vi "Correct Taus.vi"(4 "#_shots":i32=5, 6 "Filter?":bool, 8 "error in":errorcluster, 9 "filter changed?":bool, 11 "CRDS Cell in":refnum<class "CRDS Cell.lvclass">) -> (0 "error out":errorcluster, 3 "CRDS Cell out":refnum<class "CRDS Cell.lvclass">)   [LabVIEW 2014, in "CRDS Lib.lvlib" / "CRDS Cell.lvclass"]
doc: "Correct tau values for Rayleigh scattering. \n\nIf on filter:\n* The tau and tau0 values will be the uncorrected values in seconds.\n* tau0corr will be in the Rayleigh scattering corrected value in us.\n* ext, extcorr and taucorr will be set to NaN.\n\nIf on sample:\n* Tau is the raw tau value in us.\n* taucorr will be the Rayleigh scattering corrected value in us\n* ext and extCorr will be the same value."
uses:
  CRDS Cell.lvclass
  CRDS Cell.lvclass/CRDS Cell.ctl
  Data/Cell/CRDS Cell Data.lvclass/CRDS Cell Data.ctl
  Data/Cell/Read extParam.vi
  General/Atmospheric/Atmospheric Constants.vi
  Data/Cell/Read hkParam.vi
  General/Atmospheric/Atmospheric Library.lvlib
  Data/Cell/CRDS Cell Data.lvclass
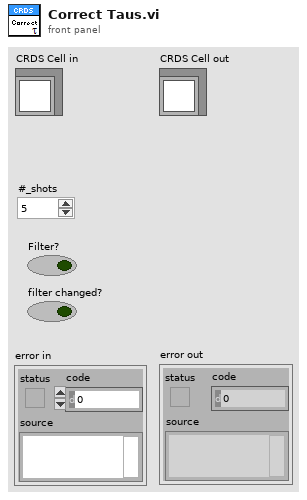
[diagram p1: front panel]
types:
  T1 = typedef "Base CRDS Lib.lvlib/calData.ctl" = cluster{"rhDilFac":sgl, "Q":sgl, "Tmean":sgl, "extDilFac":sgl, "rhCell":sgl, "P":sgl, "T":sgl}
  T2 = typedef "extparam.ctl" = cluster{"Tau":sgl, "Tau0cor":sgl, "ext":sgl, "extCorr":sgl, "stdevTau":sgl, "eTau":sgl, "taucorr":sgl, "Tau0":sgl, "max":sgl}
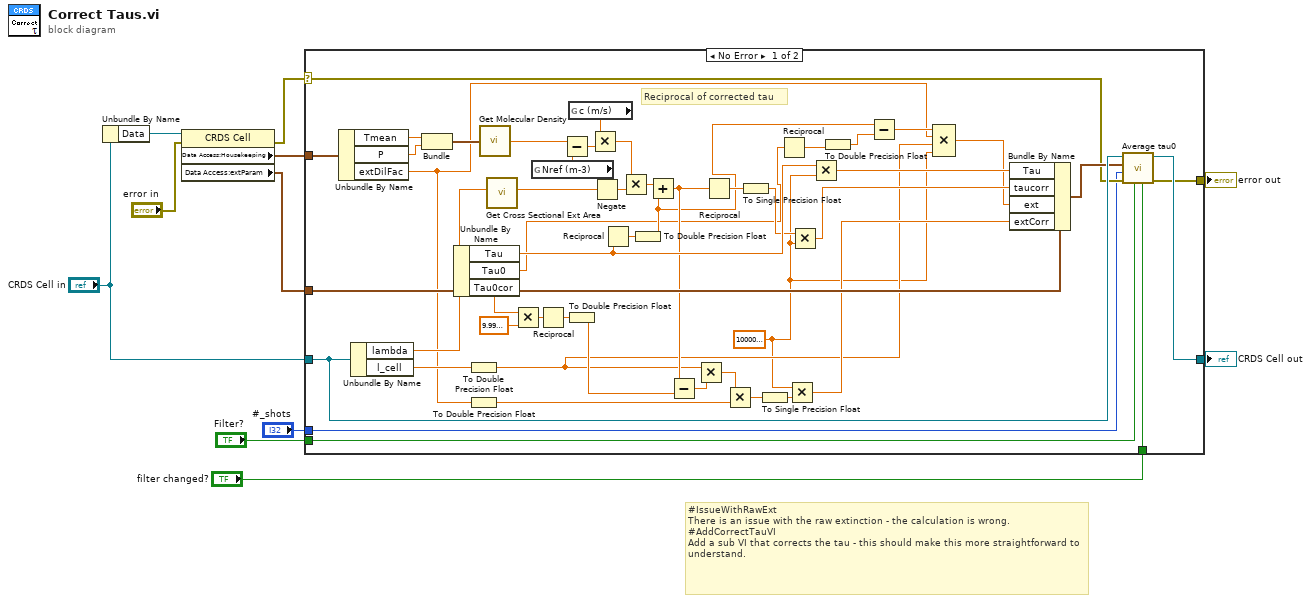
[diagram p0: block diagram]
diagram:
  # "#IssueWithRawExt\nThere is an issue with the raw extinction - the calculation is wrong.\n#AddCorrectTauVI\nAdd a sub VI that corrects the tau - this should make this more straightforward to understand."
  n1 = Unbundle By Name("CRDS Cell in") -> ("Data"=w4:refnum<class "CRDS Cell Data.lvclass">)
  n2 = property class="CRDS Cell"(reference=w4, error in="error in") -> (error out=w6:errorcluster, "Data Access:Housekeeping"=w9:T1, "Data Access:extParam"=w8:T2)  [unwired: 1 out]
  n3 = case shown="No Error" w6 {
    selector: w6 -> [w52 w63]
    tunnel: [w51 w63] -> w3
    tunnel: [w54 w62] -> w2
    tunnel: "CRDS Cell in" -> [w55 w62]
    tunnel: w9 -> [w61 _]
    tunnel: w8 -> [w59 _]
    tunnel: "Filter?" -> [w31 _]
    tunnel: "#_shots" -> [w50 _]
    tunnel: "filter changed?" -> [w49 _]
    frame No Error {
      w12 = sgl 1000000.0
      # "Reciprocal of corrected tau"
      n4 = Unbundle By Name(w61) -> ("Tmean"=w60:sgl, "P"=w56:sgl, "extDilFac"=w15:sgl)
      n5 = Unbundle By Name(w55) -> ("lambda"=w57:dbl, "l_cell"=w58:sgl)
      n6 = Bundle("Tmean"=w60, "P"=w56) -> (w29:cluster{"Tmean":sgl, "P":sgl})  [unwired: 1 in]
      n7 = Unbundle By Name(w59) -> ("Tau"=w44:sgl, "Tau0"=w16:sgl, "Tau0cor"=w21:sgl)
      n8 = To Double Precision Float(number=w58) -> (double precision float=w14:dbl)
      n9 = To Double Precision Float(number=w15) -> (double precision float=w24:dbl)
      n10 = call "Get Molecular Density.vi"("thermoCond"=w29) -> ("M (m-3)"=w30:dbl)
      n11 = call "Get Cross Sectional Ext Area.vi"("l (nm)"=w57) -> ("CAext (m2)"=w28:dbl)  [unwired: 10 in]
      n12 = Multiply(x=w21, y=sgl 1e-06) -> (x*y=w33:sgl)
      n13 = global read "Atmospheric Constants.vi" "Nref (m-3)"() -> (w48:dbl)
      n14 = Reciprocal(x=w33) -> (1/x=w34:sgl)
      n15 = Subtract(x=w30, y=w48) -> (x-y=w43:dbl)
      n16 = To Double Precision Float(number=w34) -> (double precision float=w25:dbl)
      n17 = global read "Atmospheric Constants.vi" "c (m/s)"() -> (w42:dbl)
      n18 = Multiply(x=w42, y=w43) -> (x*y=w47:dbl)
      n19 = Negate(x=w28) -> (-x=w27:dbl)
      n20 = Reciprocal(x=w44) -> (1/x=w46:sgl)
      n21 = Multiply(x=w47, y=w27) -> (x*y=w26:dbl)
      n22 = To Double Precision Float(number=w46) -> (double precision float=w18:dbl)
      n23 = Add(x=w26, y=w18) -> (x+y=w36:dbl)
      n24 = Subtract(x=w36, y=w25) -> (x-y=w40:dbl)
      n25 = Multiply(x=w14, y=w40) -> (x*y=w37:dbl)
      n26 = Reciprocal(x=w36) -> (1/x=w35:dbl)
      n27 = Multiply(x=w37, y=w24) -> (x*y=w39:dbl)
      n28 = To Single Precision Float(number=w35) -> (single precision float=w41:sgl)
      n29 = To Single Precision Float(number=w39) -> (single precision float=w38:sgl)
      n30 = Reciprocal(x=w16) -> (1/x=w20:sgl)
      n31 = Multiply(x=w12, y=w38) -> (x*y=w22:sgl)
      n32 = Multiply(x=w41, y=w12) -> (x*y=w23:sgl)
      n33 = Multiply(x=w44, y=w12) -> (x*y=w45:sgl)
      n34 = To Double Precision Float(number=w20) -> (double precision float=w19:dbl)
      n35 = Subtract(x=w18, y=w19) -> (x-y=w17:dbl)
      n36 = Compound Arithmetic op=MULTIPLY(w17, w15, w14, w12) -> (w13:dbl)
      n37 = Bundle By Name(cluster=w59, "Tau"=w45, "taucorr"=w23, "ext"=w13, "extCorr"=w22) -> (w53:T2)
      n38 = call "Average tau0.vi"("filter changed?"=w49, "filter"=w31, "error in"=w52, "# of shots"=w50, "extParam"=w53, "CRDS Cell in"=w55) -> ("error out"=w51:errorcluster, "CRDS Cell out"=w54:refnum<class "CRDS Cell.lvclass">)  [unwired: 4 in]
    }
    frame Error {
    }
  }
  "error out" <- w3
  "CRDS Cell out" <- w2
